vi "Tell Self Forward.vi"(6 "Msg":refnum<class "Msg.lvclass">, 7 "Actor in":refnum<class "Actor.lvclass">, 9 "Msg Attributes":T1 {"Teller"."Absolute Time" format="%<%x %.3X>T"}, 10 "Previous Told":bool) -> (0 "Error out":errorcluster, 1 "Told":bool, 2 "Told Or Previous Told":bool, 5 "Actor out":refnum<class "Actor.lvclass">)   [LabVIEW 2020, in "jettl.lvlib"]
uses:
  jettl.lvlib
  Actor/Actor.lvclass
  Msg Input/Msg Input.lvclass
  Msg Output/Msg Output.lvclass
  Msg/Msg.lvclass
  Relation.ctl
  Teller.ctl
  Msg Attributes.ctl
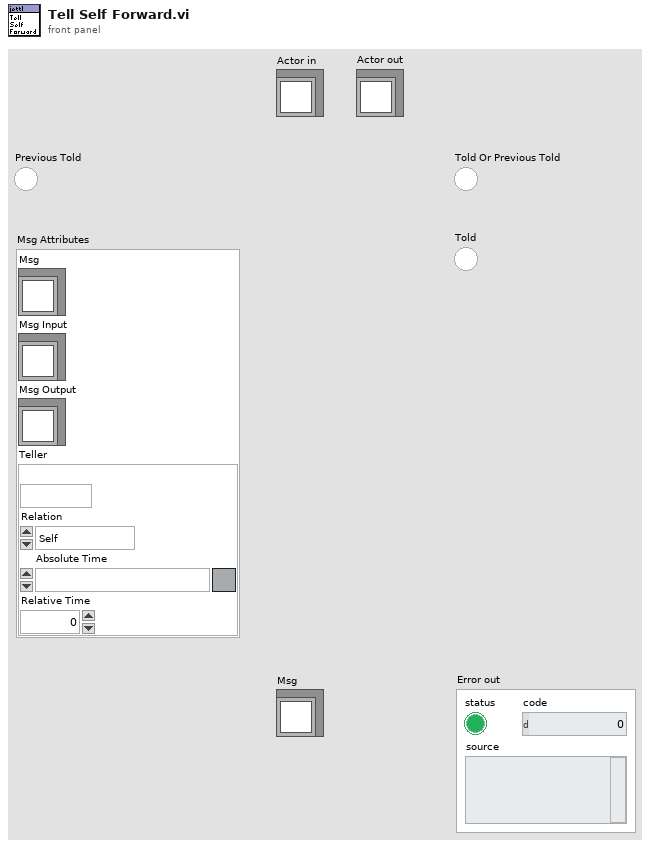
[diagram p1: front panel]
types:
  T1 = typedef "jettl.lvlib/Msg Attributes.ctl" = cluster{"Msg":refnum<class "Msg.lvclass">, "Msg Input":refnum<class "Msg Input.lvclass">, "Msg Output":refnum<class "Msg Output.lvclass">, "Teller":T2}
  T2 = typedef "jettl.lvlib/Teller.ctl" = cluster{"Alias":string, "Relation":T3, "Absolute Time":timestamp, "Relative Time":dbl}
  T3 = typedef "jettl.lvlib/Relation.ctl" = enum16{"Self", "Parent", "Child"}
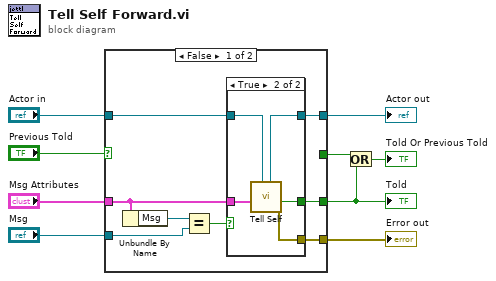
[diagram p0: block diagram]
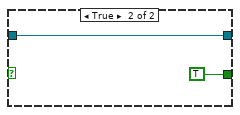
[diagram p3: hidden frame]
diagram:
  n1 = case shown="False" "Previous Told" {
    tunnel: "Actor in" -> [w17 w25]
    tunnel: [w16 _] -> w8
    tunnel: [w15 w25] -> w7
    tunnel: "Msg Attributes" -> [w12 _]
    tunnel: "Msg" -> [w11 _]
    tunnel: [w14 _] -> w1
    tunnel: [_ TRUE ("Told Or Previous Told")] -> w3
    frame False {
      n2 = Unbundle By Name(w12) -> ("Msg"=w13:refnum<class "Msg.lvclass">)
      n3 = Equal?(x=w13, y=w11) -> (x = y?=w10:bool)
      n4 = case shown="True" w10 {
        tunnel: w17 -> [w18 w22]
        tunnel: [_ w20] -> w16
        tunnel: [w18 w19] -> w15
        tunnel: w12 -> [_ w23]
        tunnel: [_ w21] -> w14
        frame False {
        }
        frame True {
          n5 = call "Tell Self.vi"("Actor in"=w22, "Msg Attributes"=w23) -> ("Error out"=w20:errorcluster, "Told"=w21:bool, "Actor out"=w19:refnum<class "Actor.lvclass">)  [unwired: 7 in]
        }
      }
    }
    frame True {
    }
  }
  "Error out" <- w8
  "Actor out" <- w7
  "Told" <- w1
  n6 = Or(x=w3, y=w1) -> (x .or. y?=→"Told Or Previous Told":bool)
